vi "MacroLoopManager_MD.vi"() -> ()   [LabVIEW 2012]
doc: "SciScan 1.2 160622"
uses:
  HFG/SubVIs/Master Slave messaging Flags.ctl
  HFG/Custom Controls and Typedefs/HB_Error Conditions Cluster.ctl
  HFG/Custom Controls and Typedefs/Heartbeat information cluster.ctl
  HFG/Custom Controls and Typedefs/Heartbeat Event Source.ctl
  Custom Controls/Heartbeat_States.ctl
  HFG/SubVIs/Heartbeat state manager Input VI names.ctl
  HFG/Custom Controls and Typedefs/HB Actionable Event.ctl
  Custom Controls and Typedefs/MacroLoopManager_STATES.ctl
  HFG/Custom Controls and Typedefs/HFG Commands.ctl
  CommonResource VIs/Timing/Timing Indicator.ctl
  CommonResource VIs/Timing/Timer Commands.ctl
  SubVIs/Macro Execution and Timing_Commands.ctl
panel:
  out "Current Execution Index":i32
  out "Master instr received":i32
  out "Slave conf received":i32
  out "Heartbeat information cluster":T1
  out "Error conditions Cluster":T4
  out "Master-Slave messaging Flags":T5={"Instruction available"=TRUE, "Slave action completed"=TRUE, "Slave Ready?"=FALSE}
  in  "stop":bool
  out "Error Out":errorcluster
  in  "Error In":errorcluster
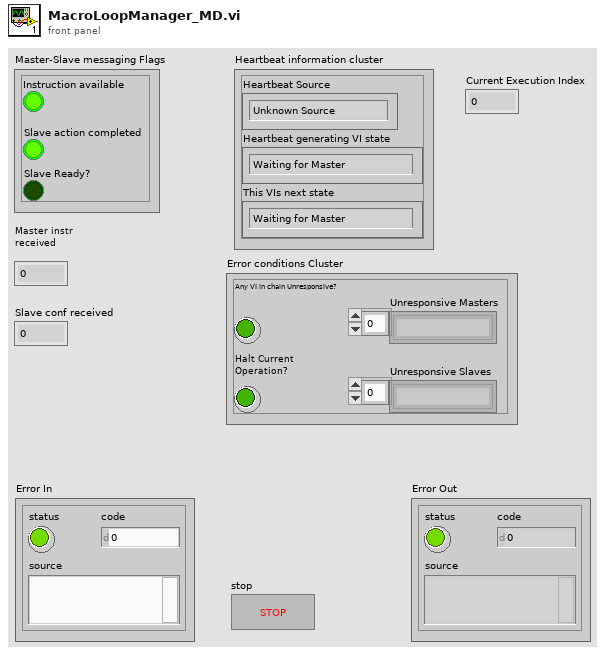
[diagram p1: front panel]
types:
  T1 = typedef "Heartbeat information cluster.ctl" = cluster{"Heartbeat Source":T2, "Heartbeat generating VI state":T3, "This VIs next state":T3}
  T2 = typedef "Heartbeat Event Source.ctl" = enum16{"Unknown Source", "Timeout", "This VI", "Master", "Slave"}
  T3 = typedef "Heartbeat_States.ctl" = enum16{"Waiting for Master", "Instruction Issued", "Waiting for Slave Completion", "Completed", "Cancelled", "Failed", "Broken Link"}
  T4 = typedef "HB_Error Conditions Cluster.ctl" = cluster{"Any VI in chain Unresponsive?":bool, "Halt Current Operation?":bool, "Unresponsive Masters":string[], "Unresponsive Slaves":string[]}
  T5 = typedef "Master Slave messaging Flags.ctl" = cluster{"Instruction available":bool, "Slave action completed":bool, "Slave Ready?":bool}
  T6 = typedef "MacroLoopManager_STATES.ctl" = enum16{"Running", "Paused", "Waiting for Trigger", "Run Preview", "Idle"}
  T7 = typedef "HB Actionable Event.ctl" = enum16{"Master instruction event", "Slave ready event", "Slave unavailable event", "Cancelled or Failed event", "Slave action complete event", "QUIT", "Broken Link", "Recovered from Broken Link"}
  T8 = typedef "Heartbeat state manager Input VI names.ctl" = cluster{"Current VI name":string, "Master VI Names":string[], "Slave VI Names":string[]}
  T9 = typedef "Macro Execution and Timing_Commands.ctl" = enum16{"Initialize (Update FGV & Rst Idx)", "Run", "EstimateTime", "Preview", "Update Macro array (Idx Unchanged)", "Update Index", "Clear Timing Info"}
  T10 = typedef "HFG Commands.ctl" = enum16{"Set", "Get", "Initialize"}
  T11 = typedef "Timing Indicator.ctl" = cluster{"Set Time":dbl, "Remaining":dbl, "Seconds":dbl, "Progress":u8, "Elapsed":dbl}
  T12 = typedef "Timer Commands.ctl" = enum16{"Clear All", "Start", "Pause", "Check Time"}
  T13 = typedef "ExecutionStatus.ctl" = enum16{"Instruction Available", "Skip", "Exec Paused", "Exec Complete", "Exec Waiting for Trigger"}
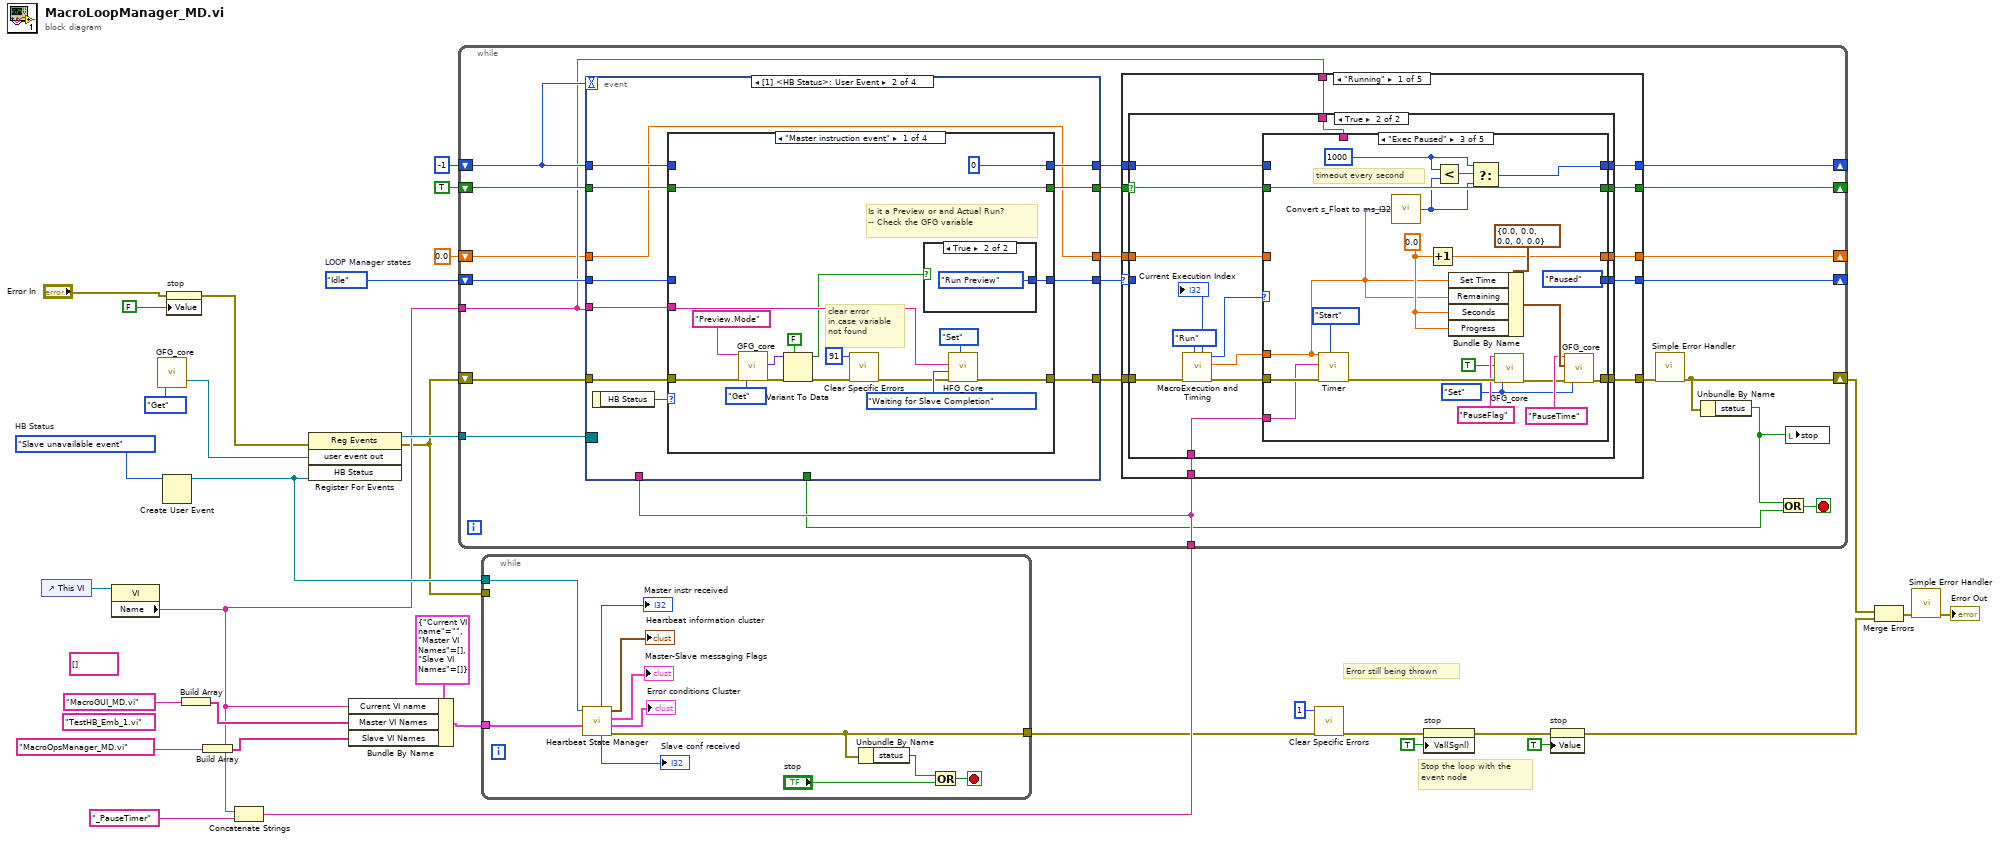
[diagram p0: block diagram]
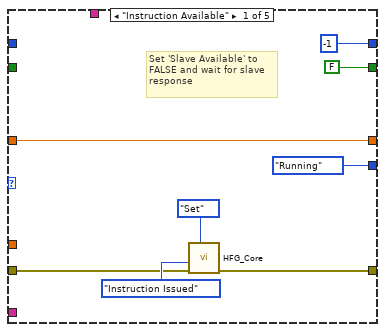
[diagram p3: hidden frame]
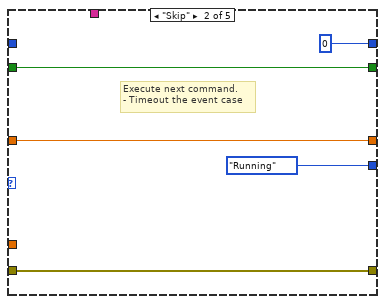
[diagram p4: hidden frame]
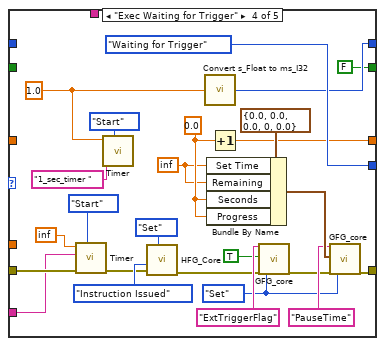
[diagram p5: hidden frame]
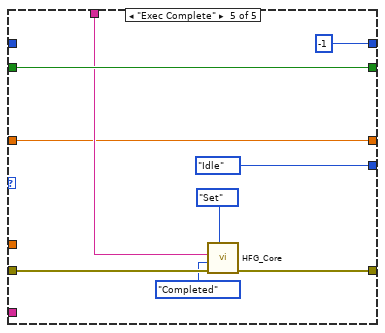
[diagram p6: hidden frame]
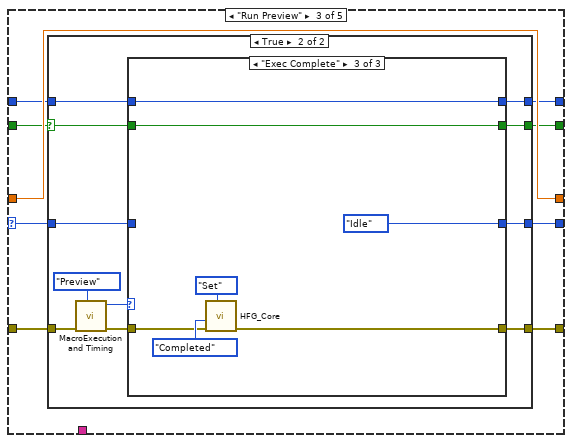
[diagram p8: hidden frame]
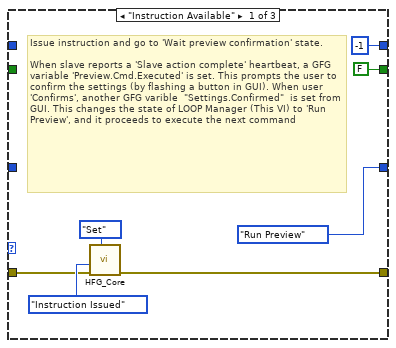
[diagram p10: hidden frame]
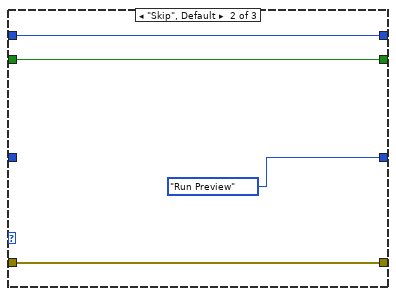
[diagram p11: hidden frame]
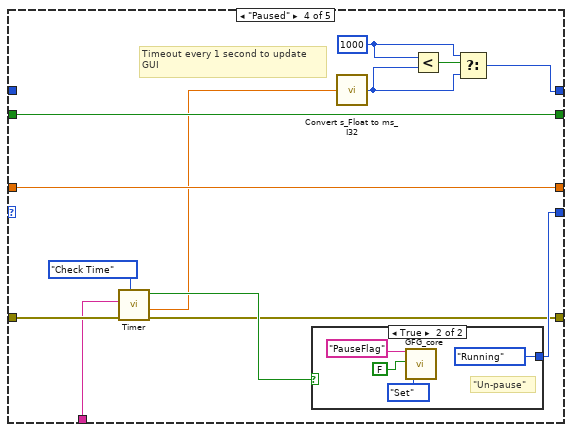
[diagram p12: hidden frame]
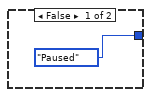
[diagram p13: hidden frame]
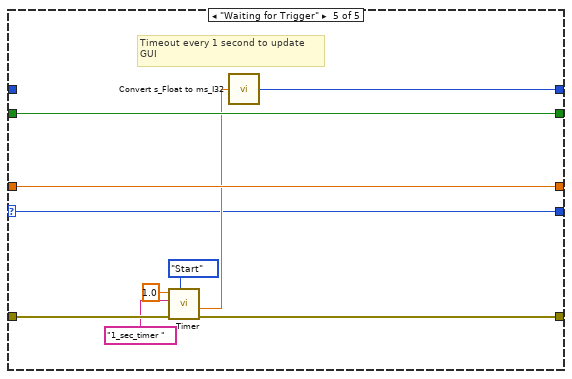
[diagram p14: hidden frame]
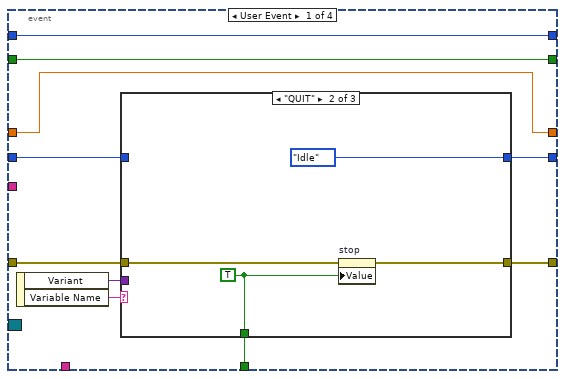
[diagram p15: hidden frame]
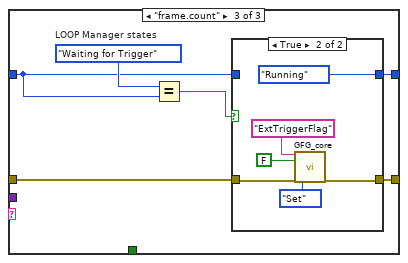
[diagram p17: hidden frame]
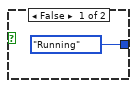
[diagram p19: hidden frame]
diagram:
  w21 = MacroLoopManager_STATES."Idle"  # LOOP Manager states
  w28 = HB_Actionable_Event."Slave unavailable event"  # HB Status
  (unwired) string[] []
  (unwired) "TestHB_Emb_1.vi"
  # "Error still being thrown"
  # "Stop the loop with the\nevent node"
  n1 = control-ref of="This VI"() -> (w31:refnum<vi>)
  n2 = property class="VI"(reference=w31) -> ("Name"=w17:string)  [unwired: 1 in, 2 out]
  n3 = call "GFG_core.vi"("Action"=enum16{"Init", "Set", "Get", "Clear"}."Get") -> ("user event out"=w29:refnum<user-event>)  [unwired: 12 in, 6 out]
  n4 = Create User Event(user event datatype=w28) -> (user event=w25:refnum<user-event>)  [unwired: 1 in, 1 out]
  n5 = property on="stop" class="Bool (strict)"(error in="Error In", "Value"=FALSE ("Stop")) -> (error out=w15:errorcluster)  [unwired: 1 in, 1 out]
  n6 = Build Array("MacroGUI_MD.vi") -> (w22:string[])
  n7 = Build Array("MacroOpsManager_MD.vi") -> (w24:string[])
  n8 = Concatenate Strings(w17, "_PauseTimer") -> (w16:string)
  n9 = register-events(error in=w15, w29, w25) -> (reference out=w26:refnum<event-registration>, error out=w8:errorcluster)  [unwired: 1 in]
  n10 = Bundle By Name(cluster=T8 {"Current VI name"="", "Master VI Names"=[], "Slave VI Names"=[]} ("Heartbeat state manager Input VI names 2"), "Current VI name"=w17, "Master VI Names"=w22, "Slave VI Names"=w24) -> (w30:T8)
  n11 = while {
    tunnel: w26 -> [w55]
    shift-right: [w34] -> w5
    shift-left: w8 -> [w54]
    tunnel: w17 -> [w43]
    shift-right: [w50] -> _
    shift-left: w21 -> [w53]
    shift-right: [w48] -> _
    shift-left: TRUE -> [w49]
    shift-right: [w46] -> _
    shift-left: -1 ("milliseconds OUT (I32)") -> [w45]
    tunnel: w16 -> [w39]
    shift-right: [w42] -> _
    shift-left: 0.0 -> [w41]
    stop <- w36 stop-if-true
    n12 = event shown="[1] <HB Status>: User Event" {
      selector: w55 -> [_ _ _ _]
      dyn-events: _ -> [_ _ _ _]
      timeout: w45 -> [_ _ _ _]
      tunnel: [w240 _ w310 _] -> w38
      tunnel: w54 -> [w239 w271 w309 w318]
      tunnel: [w238 w270 w309 w317] -> w51
      tunnel: w43 -> [_ w269 _ _]
      tunnel: [w236 w268 MacroLoopManager_STATES."Running" w319] -> w52
      tunnel: w53 -> [w237 w267 _ w319]
      tunnel: w49 -> [w235 w266 w312 w321]
      tunnel: [w235 w265 w312 w321] -> w47
      tunnel: w45 -> [w234 w264 w311 w320]
      tunnel: [w234 w263 w311 w320] -> w44
      tunnel: w41 -> [w233 w262 w308 w315]
      tunnel: [w233 w262 w308 w314] -> w40
      tunnel: w39 -> [_ _ _ w316]
      event User Event {
        n13 = event-data() -> ("Variant"=w232:variant, "Variable Name"=w241:string)  [unwired: 1 in]
        n14 = case shown="\"QUIT\"" w241 {
          tunnel: [_ w246 _] -> w240
          tunnel: [w243 w247 w250] -> w238
          tunnel: w239 -> [w243 w244 w249]
          tunnel: w237 -> [w242 _ w251]
          tunnel: [w242 MacroLoopManager_STATES."Idle" ("LOOP Manager states") w253] -> w236
          tunnel: w232 -> [_ _ _]
          frame Default {
          }
          frame "QUIT" {
            w246 = TRUE
            n15 = property on="stop" class="Bool (strict)"(error in=w244, "Value"=w246) -> (error out=w247:errorcluster)  [unwired: 1 in, 1 out]
          }
          frame "frame.count" {
            w252 = MacroLoopManager_STATES."Waiting for Trigger"  # LOOP Manager states
            n16 = Equal?(x=w252, y=w251) -> (x = y?=w248:bool)
            n17 = case shown="True" w248 {
              tunnel: [w255 MacroLoopManager_STATES."Running" ("LOOP Manager states")] -> w253
              tunnel: w249 -> [w254 w256]
              tunnel: w251 -> [w255 _]
              tunnel: [w254 w257] -> w250
              frame False {
              }
              frame True {
                n18 = call "GFG_core.vi"("Variable Name in"="ExtTriggerFlag", "Variant in"=FALSE, "error in (no error)"=w256, "Action"=enum16{"Init", "Set", "Get", "Clear"}."Set") -> ("error out"=w257:errorcluster)  [unwired: 9 in, 6 out]
              }
            }
          }
        }
      }
      event User Event {
        n19 = event-data() -> ("HB Status"=w272:T7)  [unwired: 1 in]
        n20 = case shown="\"Master instruction event\"" w272 {
          tunnel: w271 -> [w276 w295 w296 w302]
          tunnel: [w289 w295 w296 w300] -> w270
          tunnel: w269 -> [w288 _ _ _]
          tunnel: [w287 w294 w297 MacroLoopManager_STATES."Idle"] -> w268
          tunnel: w267 -> [_ w294 w297 _]
          tunnel: w266 -> [w286 w293 _ _]
          tunnel: [w286 w293 TRUE TRUE] -> w265
          tunnel: w264 -> [_ w292 w298 _]
          tunnel: [0 ("milliseconds OUT (I32)") w292 w298 -1 ("milliseconds OUT (I32)")] -> w263
          frame "Master instruction event" {
            # "clear error\nin case variable\nnot found"
            # "Is it a Preview or and Actual Run?\n-- Check the GFG variable"
            n21 = call "GFG_core.vi"("Variable Name in"="Preview.Mode", "error in (no error)"=w276, "Action"=enum16{"Init", "Set", "Get", "Clear"}."Get") -> ("Variant Out"=w278:variant, "error out"=w280:errorcluster)  [unwired: 10 in, 5 out]
            n22 = Variant To Data(error in=w280, type=FALSE, Variant=w278) -> (data=w277:bool, error out=w274:errorcluster)
            n23 = call "Clear Specific Errors.vi"("Error In"=w274, "Error number In"=91) -> ("Error Out"=w273:errorcluster)  [unwired: 8 in, 1 out]
            n24 = case shown="True" w277 {
              tunnel: [MacroLoopManager_STATES."Running" MacroLoopManager_STATES."Run Preview"] -> w287
              frame False {
              }
              frame True {
              }
            }
            n25 = call "HFG_Core.vi"("HFG Commands"=HFG_Commands."Set", "Error In"=w273, "Heartbeat state IN"=Heartbeat_States."Waiting for Slave Completion", "VI Name (Calling VIs name by default)"=w288) -> ("Error Out"=w289:errorcluster)  [unwired: 4 in, 3 out]
          }
          frame Default {
          }
          frame "Slave action complete event" {
            # "Set Slave avaiilability to TRUE.\n\nThe next commands start executing only\nif this boolean is set to TRUE"
          }
          frame "Cancelled or Failed event" {
            # "\"Un-pause\" in case cancelled occured during a pause"
            # "Reset the system"
            n26 = call "GFG_core.vi"("Variable Name in"="PauseFlag", "Variant in"=FALSE, "error in (no error)"=w302, "Action"=enum16{"Init", "Set", "Get", "Clear"}."Set") -> ("error out"=w300:errorcluster)  [unwired: 9 in, 6 out]
          }
        }
      }
      event "stop": Value Change {
        n27 = event-data() -> ("NewVal"=w310:bool)  [unwired: 1 in]
      }
      event Timeout {
        n28 = event-data() -> ()  [unwired: 1 in, 1 out]
        n29 = case shown="\"Paused\", \"Waiting for Trigger\"" w319 {
          tunnel: w318 -> [w322 w332]
          tunnel: [w323 w338] -> w314
          tunnel: w315 -> [w323 w337]
          tunnel: [w322 w336] -> w317
          tunnel: w316 -> [_ w330]
          frame Default {
          }
          frame "Paused", "Waiting for Trigger" {
            w325 = 100.0 ("y")
            # "Convert to elapsed time%"
            n30 = call "Timer.vi"("Timer Command"=Timer_Commands."Check Time", "Error In"=w332, "VI name (Optional)"=w330) -> ("Error Out"=w324:errorcluster, "Remaining Time (s)"=w329:dbl, "Elapsed Time (s)"=w328:dbl, "Set Time OUT (s)"=w327:dbl)  [unwired: 3 in, 2 out]
            n31 = Quotient & Remainder(x=w337, y=61.0) -> (x-y*floor(x/y)=w333:dbl)  [unwired: 1 out]
            n32 = Divide(x=w329, y=w327) -> (x/y=w326:dbl)
            n33 = Multiply(x=w325, y=w326) -> (x*y=w335:dbl)
            n34 = Subtract(x=w325, y=w335) -> (x-y=w334:dbl)
            n35 = Increment(x=w333) -> (x+1=w338:dbl)
            n36 = Bundle By Name(cluster=T11 {"Set Time"=0.0, "Remaining"=0.0, "Seconds"=0.0, "Progress"=0, "Elapsed"=0.0} ("Paused"), "Elapsed"=w328, "Set Time"=w327, "Remaining"=w329, "Seconds"=w333, "Progress"=w334) -> (w340:T11)
            n37 = call "GFG_core.vi"("Variable Name in"="PauseTime", "Variant in"=w340, "error in (no error)"=w324, "Action"=enum16{"Init", "Set", "Get", "Clear"}."Set") -> ("error out"=w336:errorcluster)  [unwired: 9 in, 6 out]
          }
        }
      }
    }
    n38 = case shown="\"Running\"" w52 {
      selector: w52 -> [w56 w158 w167 _ w224]
      tunnel: w51 -> [w67 w157 w169 w215 w230]
      tunnel: [w66 w158 w166 w213 w224] -> w50
      tunnel: [w65 w157 w168 w206 w228] -> w35
      tunnel: [w64 w160 w164 w212 w229] -> w48
      tunnel: w47 -> [w57 w160 w162 w212 w229]
      tunnel: [w63 w161 w163 w207 w225] -> w46
      tunnel: w44 -> [w62 w161 w165 _ _]
      tunnel: w39 -> [w61 _ _ w211 _]
      tunnel: w43 -> [w60 _ _ _ _]
      tunnel: [w59 w159 w170 w205 w227] -> w42
      tunnel: w40 -> [w58 w159 w170 w205 w227]
      frame "Running" {
        n39 = case shown="True" w57 {
          selector: w57 -> [w70 w75]
          tunnel: w67 -> [w72 w73]
          tunnel: [w71 w88] -> w66
          tunnel: [w72 w87] -> w65
          tunnel: [w70 w86] -> w64
          tunnel: [w69 w85] -> w63
          tunnel: w62 -> [w69 w84]
          tunnel: w61 -> [_ w83]
          tunnel: w60 -> [_ w82]
          tunnel: [w68 w81] -> w59
          tunnel: w58 -> [w68 w80]
          tunnel: w56 -> [w71 _]
          frame False {
          }
          frame True {
            n40 = call "MacroExecution and Timing.vi"("MacroExecution and Timing Command"=Macro_Execution_and_Timing_Commands."Run" ("MacroExecution Command"), "Error In"=w73) -> ("Error Out"=w77:errorcluster, "Pause Duration"=w78:dbl, "Execution Status"=w79:T13, "Current Execution Index"=→"Current Execution Index":i32)  [unwired: 4 in, 2 out]
            n41 = case shown="\"Exec Paused\"" w79 {
              tunnel: [MacroLoopManager_STATES."Running" ("LOOP Manager states") MacroLoopManager_STATES."Running" ("LOOP Manager states") MacroLoopManager_STATES."Paused" ("LOOP Manager states") MacroLoopManager_STATES."Waiting for Trigger" ("LOOP Manager states") MacroLoopManager_STATES."Idle" ("LOOP Manager states")] -> w88
              tunnel: w78 -> [_ _ w102 _ _]
              tunnel: w77 -> [w95 w100 w121 w146 w155]
              tunnel: [w92 w100 w117 w143 w152] -> w87
              tunnel: w75 -> [_ w99 w119 _ w151]
              tunnel: [FALSE w99 w119 FALSE w151] -> w86
              tunnel: [-1 ("milliseconds OUT (I32)") 0 ("milliseconds OUT (I32)") w106 w132 -1 ("milliseconds OUT (I32)")] -> w85
              tunnel: w84 -> [_ _ _ _ _]
              tunnel: w83 -> [_ _ w118 w144 _]
              tunnel: w82 -> [_ _ _ _ w149]
              tunnel: [w89 w97 w105 w136 w148] -> w81
              tunnel: w80 -> [w89 w97 _ _ w148]
              frame "Instruction Available" {
                # "Set 'Slave Available' to\nFALSE and wait for slave\nresponse"
                n42 = call "HFG_Core.vi"("HFG Commands"=HFG_Commands."Set", "Error In"=w95, "Heartbeat state IN"=Heartbeat_States."Instruction Issued") -> ("Error Out"=w92:errorcluster)  [unwired: 5 in, 3 out]
              }
              frame "Skip" {
                # "Execute next command.\n- Timeout the event case"
              }
              frame "Exec Paused" {
                w104 = enum16{"Init", "Set", "Get", "Clear"}."Set" ("Action")
                w109 = 1000 ("milliseconds OUT (I32)")
                w103 = 0.0 ("Seconds")
                # "timeout every second"
                n43 = call "Timer.vi"("Timer Command"=Timer_Commands."Start", "Error In"=w121, "VI name (Optional)"=w118, "Set Time IN (s)"=w102) -> ("Error Out"=w113:errorcluster)  [unwired: 2 in, 5 out]
                n44 = call "Convert s_Float to ms_I32.vi"("Seconds IN (Float)"=w102) -> ("milliseconds OUT (I32)"=w107:i32)
                n45 = Increment(x=w103) -> (x+1=w105:dbl)
                n46 = Less?(x=w109, y=w107) -> (x < y?=w108:bool)
                n47 = Bundle By Name(cluster=T11 {"Set Time"=0.0, "Remaining"=0.0, "Seconds"=0.0, "Progress"=0, "Elapsed"=0.0} ("Paused"), "Set Time"=w102, "Remaining"=w102, "Seconds"=w103, "Progress"=w103) -> (w115:T11)
                n48 = Select(t=w109, s=w108, f=w107) -> (s? t:f=w106:i32)
                n49 = call "GFG_core.vi"("Variable Name in"="PauseFlag", "Variant in"=TRUE, "error in (no error)"=w113, "Action"=w104) -> ("error out"=w110:errorcluster)  [unwired: 9 in, 6 out]
                n50 = call "GFG_core.vi"("Variable Name in"="PauseTime", "Variant in"=w115, "error in (no error)"=w110, "Action"=w104) -> ("error out"=w117:errorcluster)  [unwired: 9 in, 6 out]
              }
              frame "Exec Waiting for Trigger" {
                w124 = 1.0 ("Set Time IN (s)")
                w133 = inf
                w135 = enum16{"Init", "Set", "Get", "Clear"}."Set" ("Action")
                w134 = 0.0 ("Seconds")
                n51 = call "Timer.vi"("Timer Command"=Timer_Commands."Start", "Error In"=w146, "VI name (Optional)"=w144, "Set Time IN (s)"=inf) -> ("Error Out"=w129:errorcluster)  [unwired: 2 in, 5 out]
                n52 = call "Timer.vi"("Timer Command"=Timer_Commands."Start", "VI name (Optional)"="1_sec_timer ", "Set Time IN (s)"=w124) -> ()  [unwired: 3 in, 6 out]
                n53 = call "HFG_Core.vi"("HFG Commands"=HFG_Commands."Set", "Error In"=w129, "Heartbeat state IN"=Heartbeat_States."Instruction Issued") -> ("Error Out"=w128:errorcluster)  [unwired: 5 in, 3 out]
                n54 = call "Convert s_Float to ms_I32.vi"("Seconds IN (Float)"=w124) -> ("milliseconds OUT (I32)"=w132:i32)
                n55 = Bundle By Name(cluster=T11 {"Set Time"=0.0, "Remaining"=0.0, "Seconds"=0.0, "Progress"=0, "Elapsed"=0.0} ("Paused"), "Set Time"=w133, "Remaining"=w133, "Seconds"=w134, "Progress"=w134) -> (w141:T11)
                n56 = Increment(x=w134) -> (x+1=w136:dbl)
                n57 = call "GFG_core.vi"("Variable Name in"="ExtTriggerFlag", "Variant in"=TRUE, "error in (no error)"=w128, "Action"=w135) -> ("error out"=w137:errorcluster)  [unwired: 9 in, 6 out]
                n58 = call "GFG_core.vi"("Variable Name in"="PauseTime", "Variant in"=w141, "error in (no error)"=w137, "Action"=w135) -> ("error out"=w143:errorcluster)  [unwired: 9 in, 6 out]
              }
              frame "Exec Complete" {
                n59 = call "HFG_Core.vi"("HFG Commands"=HFG_Commands."Set", "Error In"=w155, "Heartbeat state IN"=Heartbeat_States."Completed", "VI Name (Calling VIs name by default)"=w149) -> ("Error Out"=w152:errorcluster)  [unwired: 4 in, 3 out]
              }
            }
          }
        }
      }
      frame "Idle" {
      }
      frame "Run Preview" {
        n60 = case shown="True" w162 {
          selector: w162 -> [w172 w175]
          tunnel: w169 -> [w173 w184]
          tunnel: [w173 w181] -> w168
          tunnel: w167 -> [w174 w180]
          tunnel: [w174 w179] -> w166
          tunnel: w165 -> [w171 w178]
          tunnel: [w172 w177] -> w164
          tunnel: [w171 w176] -> w163
          frame False {
          }
          frame True {
            n61 = call "MacroExecution and Timing.vi"("MacroExecution and Timing Command"=Macro_Execution_and_Timing_Commands."Preview" ("MacroExecution Command"), "Error In"=w184) -> ("Error Out"=w182:errorcluster, "Execution Status"=w183:T13)  [unwired: 4 in, 4 out]
            n62 = case shown="\"Exec Complete\"" w183 {
              tunnel: w182 -> [w190 w196 w200]
              tunnel: [w189 w196 w201] -> w181
              tunnel: w180 -> [_ _ _]
              tunnel: [MacroLoopManager_STATES."Run Preview" ("LOOP Manager states") MacroLoopManager_STATES."Run Preview" ("LOOP Manager states") MacroLoopManager_STATES."Idle" ("LOOP Manager states")] -> w179
              tunnel: w178 -> [_ w193 w197]
              tunnel: w175 -> [_ w194 w198]
              tunnel: [FALSE w194 w198] -> w177
              tunnel: [-1 ("milliseconds OUT (I32)") w193 w197] -> w176
              frame "Instruction Available" {
                # "Issue instruction and go to 'Wait preview confirmation' state.\n\nWhen slave reports a 'Slave action complete' heartbeat, a GFG variable 'Preview.Cmd.Executed' is set. This prompts the user to confirm the settings (by flashing a button in GUI). When user 'Confirms', another GFG varible  \"Settings.Confirmed\"  is set from GUI. This changes the state of LOOP Manager (This VI) to 'Run Preview', and it proceeds to execute the next command"
                n63 = call "HFG_Core.vi"("HFG Commands"=HFG_Commands."Set", "Error In"=w190, "Heartbeat state IN"=Heartbeat_States."Instruction Issued") -> ("Error Out"=w189:errorcluster)  [unwired: 5 in, 3 out]
              }
              frame "Skip", Default {
              }
              frame "Exec Complete" {
                n64 = call "HFG_Core.vi"("HFG Commands"=HFG_Commands."Set", "Error In"=w200, "Heartbeat state IN"=Heartbeat_States."Completed") -> ("Error Out"=w201:errorcluster)  [unwired: 5 in, 3 out]
              }
            }
          }
        }
      }
      frame "Paused" {
        w209 = 1000 ("milliseconds OUT (I32)")
        # "Timeout every 1 second to update \nGUI"
        n65 = call "Timer.vi"("Timer Command"=Timer_Commands."Check Time", "Error In"=w215, "VI name (Optional)"=w211) -> ("Error Out"=w206:errorcluster, "Remaining Time (s)"=w204:dbl, "Complete?"=w214:bool)  [unwired: 3 in, 3 out]
        n66 = case shown="True" w214 {
          tunnel: [MacroLoopManager_STATES."Paused" MacroLoopManager_STATES."Running"] -> w213
          frame False {
          }
          frame True {
            # "\"Un-pause\""
            n67 = call "GFG_core.vi"("Variable Name in"="PauseFlag", "Variant in"=FALSE, "Action"=enum16{"Init", "Set", "Get", "Clear"}."Set") -> ()  [unwired: 10 in, 7 out]
          }
        }
        n68 = call "Convert s_Float to ms_I32.vi"("Seconds IN (Float)"=w204) -> ("milliseconds OUT (I32)"=w208:i32)
        n69 = Less?(x=w209, y=w208) -> (x < y?=w210:bool)
        n70 = Select(t=w209, s=w210, f=w208) -> (s? t:f=w207:i32)
      }
      frame "Waiting for Trigger" {
        # "Timeout every 1 second to update \nGUI"
        n71 = call "Timer.vi"("Timer Command"=Timer_Commands."Start", "Error In"=w230, "VI name (Optional)"="1_sec_timer ", "Set Time IN (s)"=1.0) -> ("Error Out"=w228:errorcluster, "Remaining Time (s)"=w226:dbl)  [unwired: 2 in, 4 out]
        n72 = call "Convert s_Float to ms_I32.vi"("Seconds IN (Float)"=w226) -> ("milliseconds OUT (I32)"=w225:i32)
      }
    }
    n73 = call <vilib>:"Simple Error Handler.vi"("error in (no error)"=w35) -> ("error out"=w34:errorcluster)  [unwired: 4 in, 4 out]
    n74 = Unbundle By Name(w34) -> ("status"=w37:bool)
    n75 = Or(x=w37, y=w38) -> (x .or. y?=w36:bool)
    n76 = local write "stop"(w37) -> ()
  }
  n77 = while {
    tunnel: w30 -> [w349]
    tunnel: w25 -> [w348]
    tunnel: [w344] -> w12
    tunnel: w8 -> [_]
    stop <- w346 stop-if-true
    n78 = call "Heartbeat State Manager.vi"("Heartbeat state manager Input VI names"=w349, "HB Command Event IN"=w348) -> ("Error Out"=w344:errorcluster, "Error conditions Cluster"=→"Error conditions Cluster":T4, "Master-Slave messaging Flags"=→"Master-Slave messaging Flags":T5, "Heartbeat information cluster"=→"Heartbeat information cluster":T1, "Slave Completions Received"=→"Slave conf received":i32, "Master Instructions Issued"=→"Master instr received":i32)  [unwired: 4 in]
    n79 = Unbundle By Name(w344) -> ("status"=w345:bool)
    n80 = Or(x=w345, y="stop") -> (x .or. y?=w346:bool)
  }
  n81 = call "Clear Specific Errors.vi"("Error In"=w12, "Error number In"=1) -> ("Error Out"=w10:errorcluster)  [unwired: 8 in, 1 out]
  n82 = property on="stop" class="Bool (strict)"(error in=w10, "Val(Sgnl)"=TRUE ("Value (Signaling)")) -> (error out=w7:errorcluster)  [unwired: 1 in, 1 out]
  n83 = property on="stop" class="Bool (strict)"(error in=w7, "Value"=TRUE ("stop")) -> (error out=w4:errorcluster)  [unwired: 1 in, 1 out]
  n84 = Merge Errors(w5, w4) -> (w1:errorcluster)
  n85 = call <vilib>:"Simple Error Handler.vi"("error in (no error)"=w1) -> ("error out"=→"Error Out":errorcluster)  [unwired: 4 in, 4 out]
